vi "Convert_to_2009.vi"(8 "error in (no error)":errorcluster, 11 "IB_RegDest_Label in":refnum<class "IB_RegDest_Label.lvclass">) -> (0 "error out":errorcluster, 2 "preserve?":bool, 3 "RegDest":T1)   [LabVIEW 2020, in "IB_RegDest_Label.lvclass"]
uses:
  <vilib>/AppBuilder/IB_Classes/RegDest/RegDest_Label/IB_RegDest_Label.lvclass
  <vilib>/AppBuilder/IB_Classes/RegDest/RegDest_Label/IB_RegDest_Label.lvclass/IB_RegDest_Label.ctl
  <resource>/Framework/Providers/Builds/Installer/CDK_sTypeDef_DirInfo.ctl
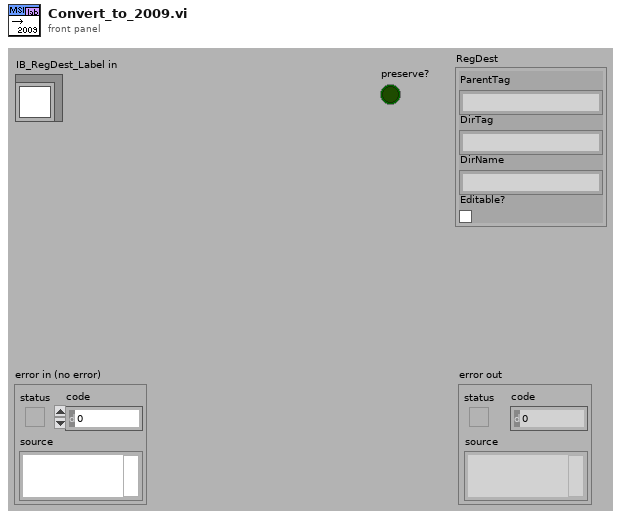
[diagram p1: front panel]
types:
  T1 = typedef "CDK_sTypeDef_DirInfo.ctl" = cluster{"ParentTag":string, "DirTag":string, "DirName":string, "Editable?":bool}
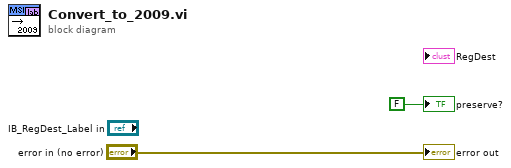
[diagram p0: block diagram]
diagram:
  "error out" <- "error in (no error)"
  "preserve?" <- FALSE ("preserve?")
